vi "UIRef.vi"(8 "error in":errorcluster, 11 "Engine in":refnum<class "Engine Parent Editor Node.lvclass">) -> (0 "error out":errorcluster, 2 "VI refnum":refnum<vi>, 3 "Engine out":refnum<class "Engine Parent Editor Node.lvclass">)   [LabVIEW 2013, in "PL Framework Configuration Tool.lvlib" / "Engine Parent Editor Node.lvclass"]
doc: "Stores the static reference to the UI of the node."
uses:
  Engine Parent Editor Node.lvclass
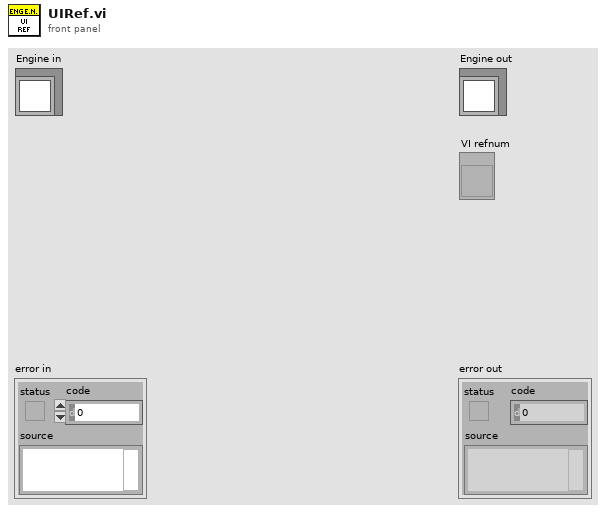
[diagram p1: front panel]
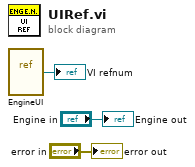
[diagram p0: block diagram]
diagram:
  n1 = vi-ref "EngineUI.vi"() -> (→"VI refnum":refnum<vi>)
  "error out" <- "error in"
  "Engine out" <- "Engine in"
